vi "Untitled 1.vi"() -> ()   [LabVIEW 2015]
uses:
  <vilib>/myRIO/Instrument Drivers/Onboard IO/DIO/DIO.lvlib
panel:
  in  "reversed array":bool[](array[boolean])
  out "number":i32 format="%b"
  out "Numeric 3":i32=8388607 format="%b"
  out "Waveform Chart":i16(graph)
  in  "A/DIO9 (Pin 13)":bool
  out "A/DIO0 (Pin 11)":bool
  in  "stop":bool
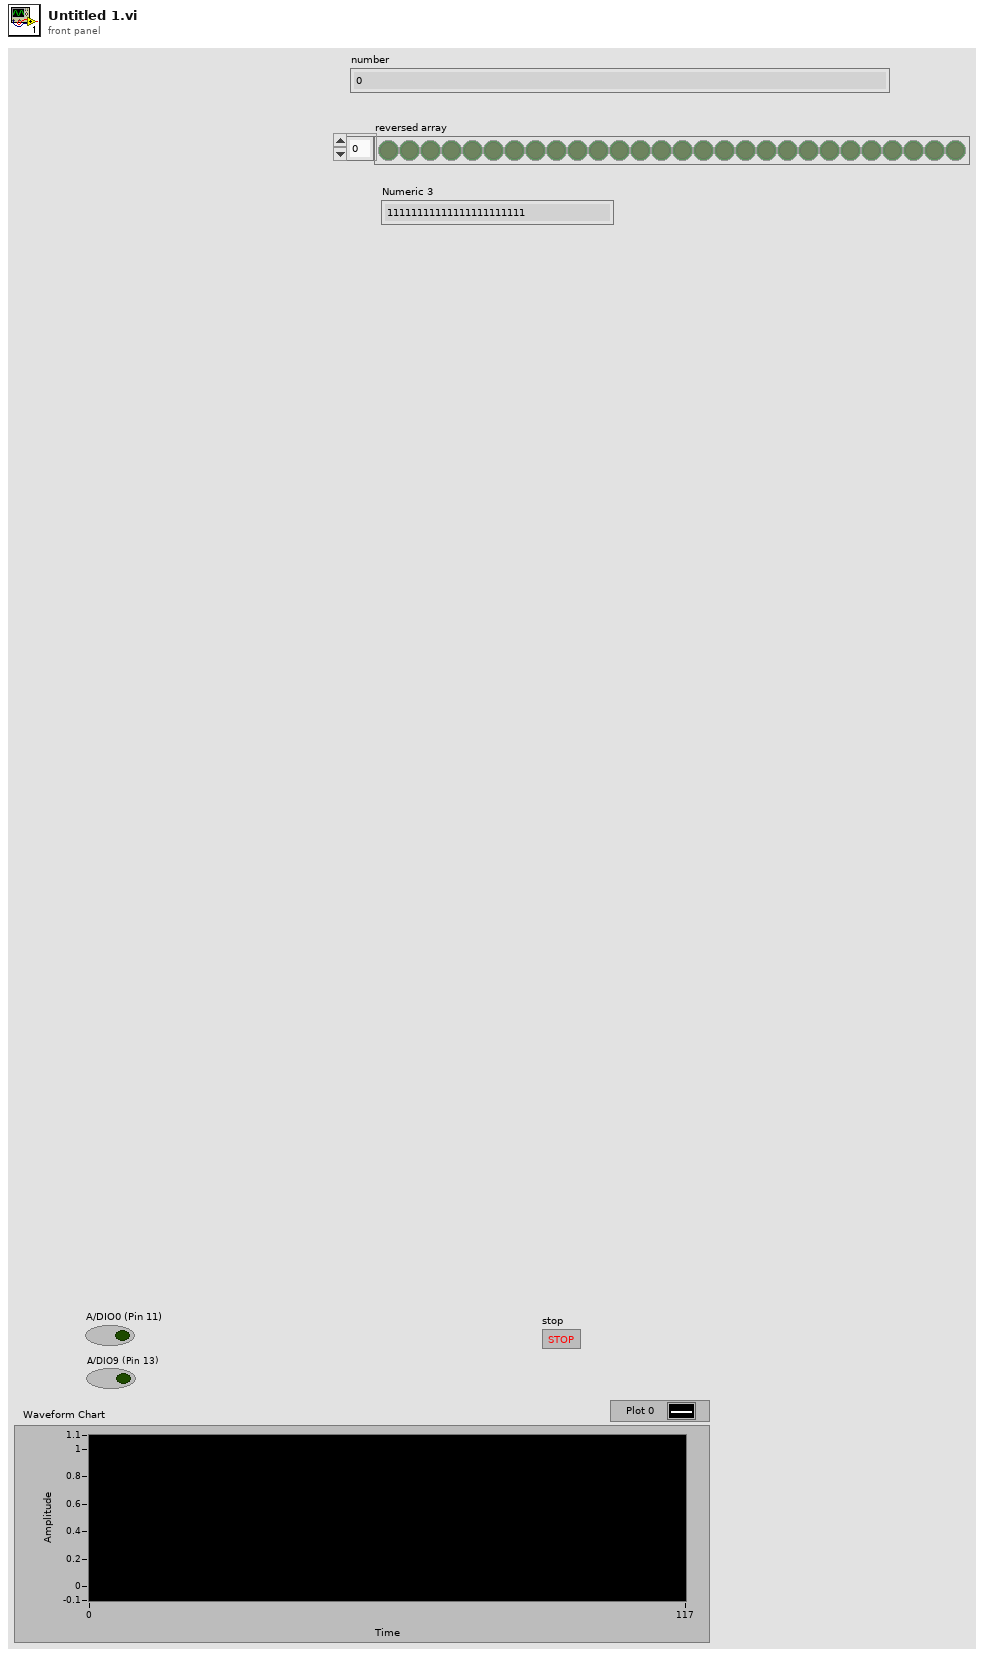
[diagram p1: front panel]
types:
  T1 = typedef "DIO.lvlib/DIO Reference.ctl" = cluster{"myRIO Reference":T2, "DIO Channels List":T6}
  T2 = typedef "myRIO Generic Hardware Reference.ctl" = cluster{"myRIO Model":T3, "myRIO Hardware Reference":T4}
  T3 = typedef "Hardware Version Enum.ctl" = enum16{"Unknown", "myRIO-1900", "myRIO-1950", "roboRIO"}
  T4 = typedef "myRIO v1.0 Reference.ctl" = cluster{"Generic FPGA Reference":T5, "Allow multiple opens":bool}
  T5 = typedef "Generic FPGA Reference.ctl" = refnum<k20>
  T6 = typedef "DIO Channels List.ctl" = T7[]
  T7 = typedef "DIO Channels Enum.ctl" = enum16{"Not Connected", "C/DIO0", "C/DIO1", "C/DIO2", "C/DIO3", "C/DIO4", "C/DIO5", "C/DIO6", "C/DIO7", "A/DIO0", "A/DIO1", "A/DIO2", "A/DIO3", "A/DIO4", "A/DIO5", "A/DIO6", "A/DIO7", "A/DIO8", "A/DIO9", "A/DIO10", "A/DIO11", "A/DIO12", "A/DIO13", "A/DIO14", "A/DIO15", "B/DIO0", "B/DIO1", "B/DIO2", "B/DIO3", "B/DIO4", "B/DIO5", "B/DIO6", "B/DIO7", "B/DIO8", "B/DIO9", "B/DIO10", "B/DIO11", "B/DIO12", "B/DIO13", "B/DIO14", "B/DIO15", "LED0", "LED1", "LED2", "LED3", "Button0", "DIO/DIO0", "DIO/DIO1", "DIO/DIO2", "DIO/DIO3", "DIO/DIO4", "DIO/DIO5", "DIO/DIO6", "DIO/DIO7", "DIO/DIO8", "DIO/DIO9", "SPI/CS0", "SPI/CS1", "SPI/CS2", "SPI/CS3", "LED RADIO (Green)", "LED RADIO (Red)", "LED COMM (Green)", "LED COMM (Red)", "LED MODE (Green)", "LED MODE (Red)"}
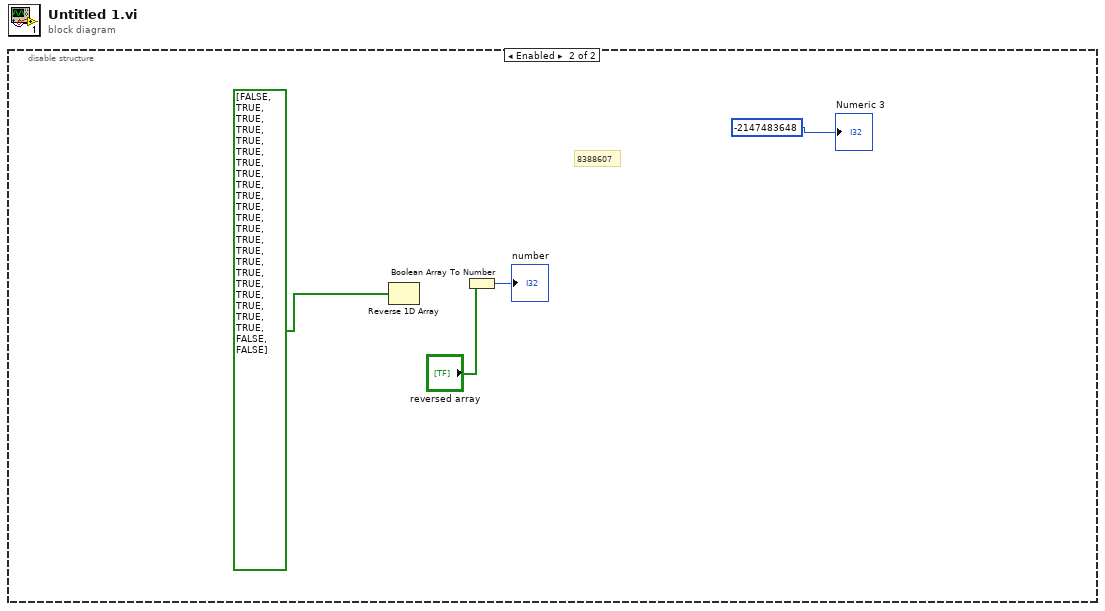
[diagram p0: block diagram]
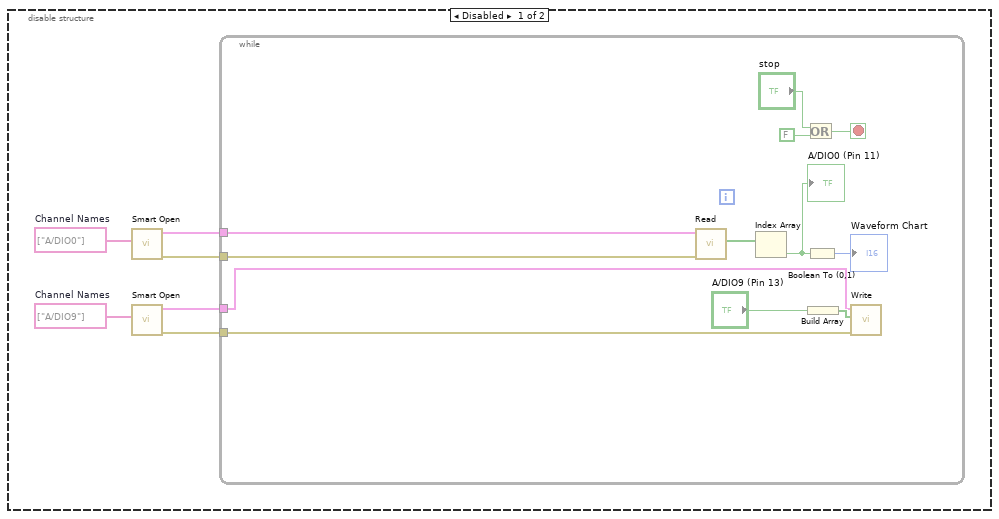
[diagram p2: hidden frame]
diagram:
  n1 = disable-structure shown="Enabled" {
    frame Disabled {
      w3 = tag[] ["A/DIO9"]  # Channel Names
      w6 = tag[] ["A/DIO0"]  # Channel Names
      n2 = call <vilib>:"Smart Open.vi"("Channel Names"=w6) -> ("error out"=w4:errorcluster, "DIO Ref Out"=w5:T1)  [unwired: 9 in]
      n3 = call <vilib>:"Smart Open.vi"("Channel Names"=w3) -> ("error out"=w1:errorcluster, "DIO Ref Out"=w2:T1)  [unwired: 9 in]
      n4 = while {
        tunnel: w5 -> [w17]
        tunnel: w4 -> [w16]
        tunnel: w2 -> [w13]
        tunnel: w1 -> [w12]
        stop <- w8 stop-if-true
        n5 = call <vilib>:"Read.vi"("error in (no error)"=w16, "DIO Ref In"=w17) -> ("Values"=w18:bool[])  [unwired: 7 in, 2 out]
        n6 = Index Array(array=w18) -> (element=w11:bool)  [unwired: 1 in]
        "A/DIO0 (Pin 11)" <- w11
        n7 = Or(x="stop", y=FALSE) -> (x .or. y?=w8:bool)
        n8 = Boolean To (0,1)(Boolean=w11) -> (0, 1=→"Waveform Chart":i16)
        n9 = Build Array("A/DIO9 (Pin 13)") -> (w14:bool[])
        n10 = call <vilib>:"Write.vi"("error in (no error)"=w12, "Values"=w14, "DIO Ref In"=w13) -> ()  [unwired: 6 in, 2 out]
      }
    }
    frame Enabled {
      # "8388607"
      n11 = Reverse 1D Array(array=bool[] [FALSE, TRUE, TRUE, TRUE, TRUE, TRUE, TRUE, TRUE, TRUE, TRUE, TRUE, TRUE, TRUE, TRUE, TRUE, TRUE, TRUE, TRUE, TRUE, TRUE, TRUE, TRUE, FALSE, FALSE]) -> ()  [unwired: 1 out]
      n12 = Boolean Array To Number(Boolean array="reversed array") -> (number=→"number":i32)
      "Numeric 3" <- -2147483648
    }
  }
